vi "Circular Data Buffer Filtered.vi"(4 "Row Size":u32=55, 6 "Buffer Size":u32=1000, 7 "Data In":dbl[][](array[numeric]), 9 "Read Size":u32, 10 "Read Location":i32, 11 "Action":enum16{"Initialize", "Write", "Read", "Clear"}(ring)) -> (1 "Buffer Size":u32, 2 "Data Out":dbl[][](array[numeric]), 3 "Next Write":u32)   [LabVIEW 2020]
doc: "Author: Scott Hannahs <sth@magnet.fsu.edu>\nCopyright 2018 Florida State University, All rights reserved."
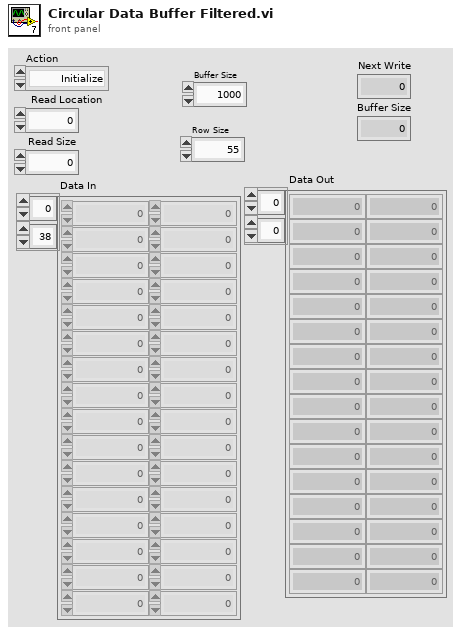
[diagram p1: front panel]
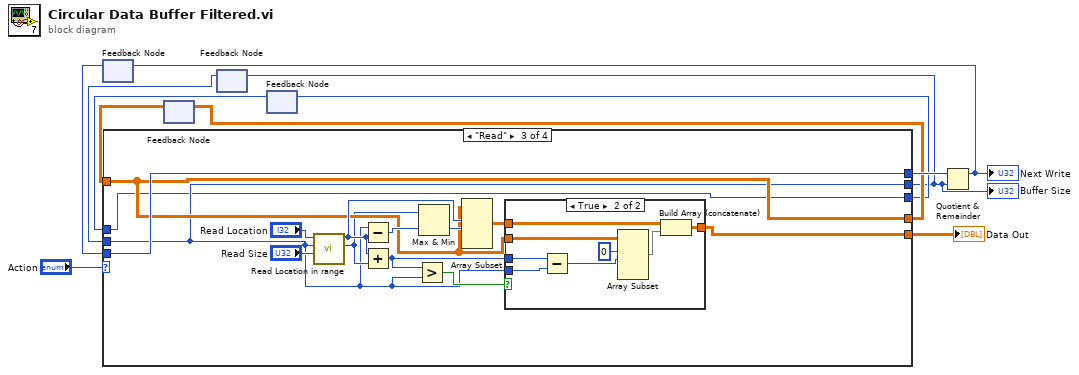
[diagram p0: block diagram]
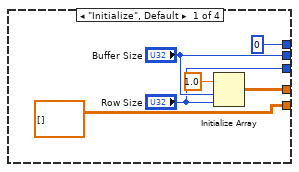
[diagram p2: hidden frame]
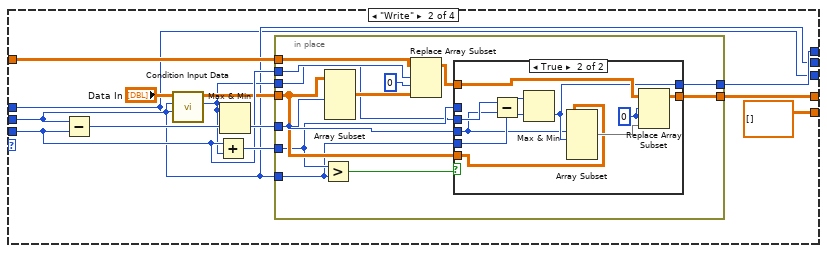
[diagram p3: hidden frame]
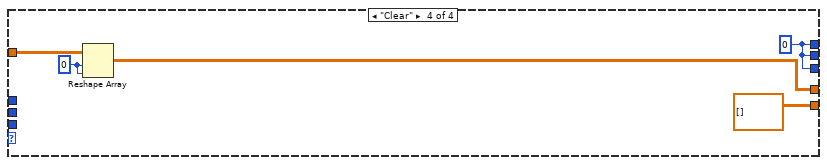
[diagram p6: hidden frame]
diagram:
  n1 = feedback #1() -> (w6:u32)  [unwired: 1 in]
  n2 = feedback #2() -> (w10:dbl[][])  [unwired: 1 in]
  n3 = feedback #3() -> (w5:u32)  [unwired: 1 in]
  n4 = feedback #4() -> (w3:u32)  [unwired: 1 in]
  n5 = case shown="\"Read\"" "Action" {
    tunnel: w5 -> [_ w20 w58 _]
    tunnel: [w16 w24 w62 w81] -> w7
    tunnel: w10 -> [_ w23 w62 w82]
    tunnel: [u32 0 w29 w69 w80] -> w8
    tunnel: w6 -> [_ w25 w69 _]
    tunnel: ["Buffer Size" w20 w58 w80] -> w2
    tunnel: ["Row Size" w19 w57 w80] -> w4
    tunnel: w3 -> [_ w19 w57 _]
    tunnel: [dbl[][] [] dbl[][] [] w56 dbl[][] []] -> w1
    frame "Initialize", Default {
      n6 = Initialize Array(1.0, "Buffer Size", "Row Size") -> (w16:dbl[][])
    }
    frame "Write" {
      n7 = Subtract(x=w20, y=w25) -> (x-y=w30:u32)
      n8 = call "Condition Input Data.vi"("Data Size"=w19, "Circular Buffer Size"=w20, "Data In"="Data In") -> ("Input Data Size"=w21:u32, "Data In Conditioned"=w22:dbl[][])  [unwired: 7 in]
      n9 = Add(x=w25, y=w21) -> (x+y=w26:u32)
      n10 = Max & Min(x=w21, y=w30) -> (min(x,y)=w28:u32)  [unwired: 1 out]
      n11 = in-place {
        in-place-border: [w39] -> w29
        in-place-border: w28 -> [w38]
        in-place-border: w22 -> [w37]
        in-place-border: w26 -> [w36]
        in-place-border: w25 -> [w35]
        in-place-border: w20 -> [w34]
        in-place-border: w21 -> [w33]
        in-place-border: [w32] -> w24
        in-place-border: w23 -> [w31]
        n12 = Greater?(x=w36, y=w34) -> (0:w41:bool)
        n13 = Array Subset(array=w37, length (row)=w38) -> (w42:dbl[][])  [unwired: 3 in]
        n14 = Replace Array Subset(array=w31, new element=w42, index (row)=w35, index (col)=0 ("disabled index (col)")) -> (w40:dbl[][])
        n15 = case shown="True" w41 {
          tunnel: w40 -> [w45 w54]
          tunnel: [w45 w55] -> w32
          tunnel: [w44 w50] -> w39
          tunnel: w36 -> [w44 _]
          tunnel: w38 -> [_ w46]
          tunnel: w37 -> [_ w51]
          tunnel: w34 -> [_ w49]
          tunnel: w33 -> [_ w47]
          frame False {
          }
          frame True {
            w53 = 0 ("index (row)")
            n16 = Subtract(x=w47, y=w46) -> (x-y=w48:u32)
            n17 = Max & Min(x=w48, y=w49) -> (min(x,y)=w50:u32)  [unwired: 1 out]
            n18 = Array Subset(array=w51, index (row)=w46, length (row)=w50) -> (w52:dbl[][])  [unwired: 2 in]
            n19 = Replace Array Subset(array=w54, new element=w52, index (row)=w53, index (col)=w53) -> (w55:dbl[][])
          }
        }
      }
    }
    frame "Read" {
      n20 = call "Read Location in range.vi"("Read Size"="Read Size", "Circular Buffer Size"=w58, "Read Location"="Read Location") -> ("Corrected Read Size"=w59:u32, "Corrected Read Locaton"=w66:u32)  [unwired: 7 in]
      n21 = Subtract(x=w58, y=w66) -> (x-y=w65:u32)
      n22 = Add(x=w66, y=w59) -> (x+y=w61:u32)
      n23 = Greater?(x=w61, y=w58) -> (0:w63:bool)
      n24 = Max & Min(x=w59, y=w65) -> (min(x,y)=w67:u32)  [unwired: 1 out]
      n25 = Array Subset(array=w62, index (row)=w66, length (row)=w67) -> (w64:dbl[][])  [unwired: 2 in]
      n26 = case shown="True" w63 {
        tunnel: w64 -> [w70 w77]
        tunnel: w62 -> [_ w76]
        tunnel: [w70 w74] -> w56
        tunnel: w58 -> [_ w72]
        tunnel: w61 -> [_ w71]
        frame False {
        }
        frame True {
          n27 = Subtract(x=w71, y=w72) -> (x-y=w73:u32)
          n28 = Array Subset(array=w76, index (row)=0 ("index"), length (row)=w73) -> (w78:dbl[][])  [unwired: 2 in]
          n29 = Build Array (concatenate)(w77, w78) -> (w74:dbl[][])
        }
      }
    }
    frame "Clear" {
      w80 = u32 0
      w83 = 0 ("dimension size")
      n30 = Reshape Array(w82, w83, w83) -> (w81:dbl[][])
    }
  }
  "Buffer Size" <- w2
  "Data Out" <- w1
  n31 = feedback-in #2(w7) -> ()
  n32 = feedback-in #3(w2) -> ()
  n33 = feedback-in #4(w4) -> ()
  n34 = Quotient & Remainder(x=w8, y=w2) -> (x-y*floor(x/y)=w9:u32)  [unwired: 1 out]
  "Next Write" <- w9
  n35 = feedback-in #1(w9) -> ()
